vi "Read U24.vi"(0 "I2C In":refnum<class "I2C.lvclass">, 1 "Slave Address":u8, 5 "Register":u32, 11 "Error In":errorcluster, 12 "Register Size":T2, 13 "Byte Order":T1) -> (4 "I2C Out":refnum<class "I2C.lvclass">, 6 "Value":u32, 15 "Error Out":errorcluster)   [LabVIEW 2020, in "lv_i2c_hal.lvlib" / "I2C.lvclass"]
uses:
  I2C.lvclass
  Register Address Size.ctl
  Byte Order.ctl
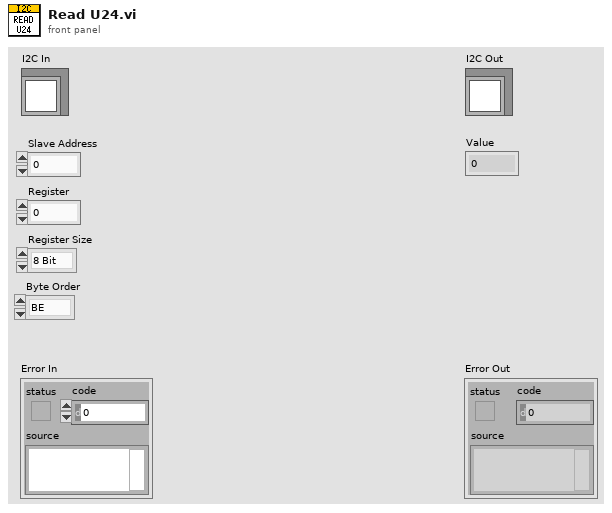
[diagram p1: front panel]
types:
  T1 = typedef "lv_i2c_hal.lvlib/I2C.lvclass/Byte Order.ctl" = enum16{"BE", "LE"}
  T2 = typedef "lv_i2c_hal.lvlib/I2C.lvclass/Register Address Size.ctl" = enum16{"8 Bit", "16 Bit", "24 Bit", "32 Bit"}
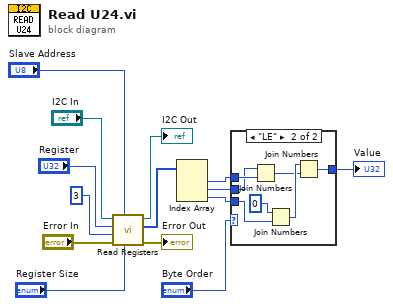
[diagram p0: block diagram]
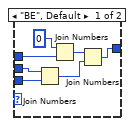
[diagram p2: hidden frame]
diagram:
  n1 = call "Read Registers.vi"("Register Size"="Register Size", "Slave Address"="Slave Address", "Error In"="Error In", "Count"=3, "Register"="Register", "I2C In"="I2C In") -> ("Error Out"=→"Error Out":errorcluster, "Values"=w11:u8[], "I2C Out"=→"I2C Out":refnum<class "I2C.lvclass">)  [unwired: 3 in]
  n2 = Index Array(array=w11) -> (element #1=w8:u8, element #2=w7:u8, element #3=w1:u8)  [unwired: 3 in]
  n3 = case shown="\"LE\"" "Byte Order" {
    tunnel: w8 -> [w19 w28]
    tunnel: w7 -> [w18 w27]
    tunnel: [w16 w22] -> w6
    tunnel: w1 -> [w17 w26]
    frame "BE", Default {
      n4 = Join Numbers(hi=w18, lo=w17) -> ((hi.lo)=w20:u16)
      n5 = Join Numbers(hi=u8 0, lo=w19) -> ((hi.lo)=w21:u16)
      n6 = Join Numbers(hi=w21, lo=w20) -> ((hi.lo)=w16:u32)
    }
    frame "LE" {
      n7 = Join Numbers(hi=w27, lo=w28) -> ((hi.lo)=w23:u16)
      n8 = Join Numbers(hi=u8 0, lo=w26) -> ((hi.lo)=w24:u16)
      n9 = Join Numbers(hi=w24, lo=w23) -> ((hi.lo)=w22:u32)
    }
  }
  "Value" <- w6
